vi "MVE Is FXP TD.vi"(11 "TD":u8[](array[numeric])) -> (3 "Boolean":bool=TRUE)   [LabVIEW 2016]
uses:
  <vilib>/variable/Type Descriptor.ctl
  <vilib>/Utility/VariantDataType/VariantType.lvlib
  <vilib>/variable/NI_Variable.lvlib
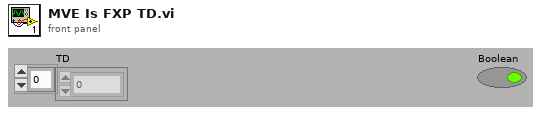
[diagram p1: front panel]
types:
  T1 = typedef "NI_Variable.lvlib/Type Descriptor.ctl" = cluster{"Variant":variant}
  T2 = typedef "VariantType.lvlib/Type.ctl" = enum8{"Invalid Type", "Void", "I8", "I16", "I32", "I64", "U8", "U16", "U32", "U64", "Single Float", "Double Float", "Extended Float", "Single Complex", "Double Complex", "Extended Complex", "Enum U8", "Enum U16", "Enum U32", "Enum U64", "Single Float With Unit", "Double Float With Unit", "Extended Float With Unit", "Single Complex with Unit", "Double Complex with Unit", "Extended Complex with Unit", "Boolean", "String", "Path", "Picture", "Tag", "Array", "Cluster", "Variant", "LV Variant", "Waveform", "Timestamp", "Digital Waveform", "Digital Data", "ExpressData", "Refnum", "External Data", "VI", "Poly VI", "LabVIEW Class Instance", "Fixed Point"}
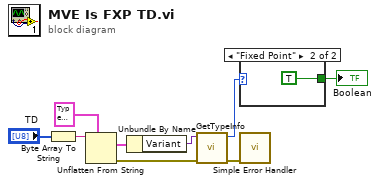
[diagram p0: block diagram]
diagram:
  n1 = Byte Array To String(unsigned byte array="TD") -> (string=w8:string)
  n2 = Unflatten From String(type=T1 {"Variant"=variant} ("type descriptor"), binary string=w8) -> (value=w7:T1, error out=w6:errorcluster)  [unwired: 3 in, 1 out]
  n3 = Unbundle By Name(w7) -> ("Variant"=w5:variant)
  n4 = call <vilib>:"GetTypeInfo.vi"("error in (no error)"=w6, "Variant"=w5) -> ("error out"=w1:errorcluster, "Type Enum"=w3:T2)  [unwired: 8 out]
  n5 = case shown="\"Fixed Point\"" w3 {
    tunnel: [_ TRUE] -> w2
    frame "Invalid Type", Default {
    }
    frame "Fixed Point" {
    }
  }
  "Boolean" <- w2
  n6 = call <vilib>:"Simple Error Handler.vi"("error in (no error)"=w1) -> ()  [unwired: 4 in, 5 out]
